vi "copy template project.vi"(8 "error in":errorcluster, 11 "project directory":path) -> (0 "error out":errorcluster)   [LabVIEW 2014, in "CD model script.lvlib"]
uses:
  CD model script.lvlib
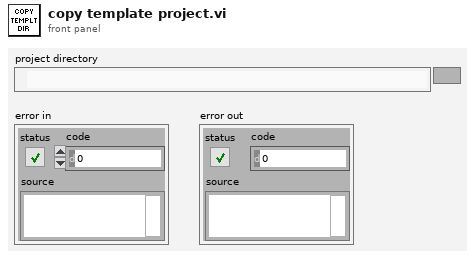
[diagram p1: front panel]
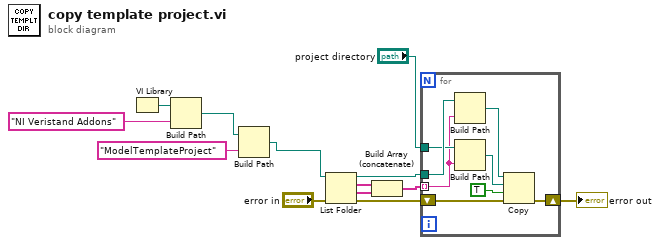
[diagram p0: block diagram]
diagram:
  n1 = VI Library() -> (path=w1:path)
  n2 = Build Path(base path=w1, name or relative path="NI Veristand Addons") -> (appended path=w3:path)
  n3 = Build Path(base path=w3, name or relative path="ModelTemplateProject") -> (appended path=w10:path)
  n4 = List Folder(path=w10, error in="error in") -> (path out=w8:path, filenames=w7:string[], folder names=w6:string[], error out=w9:errorcluster)  [unwired: 2 in]
  n5 = Build Array (concatenate)(w7, w6) -> (w5:string[])
  n6 = for {
    tunnel: "project directory" -> [w17]
    shift-right: [w20] -> w13
    shift-left: w9 -> [w21]
    tunnel: w8 -> [w18]
    tunnel: w5 -> [w16] mode=indexing
    n7 = Build Path(base path=w18, name or relative path=w16) -> (appended path=w14:path)
    n8 = Build Path(base path=w17, name or relative path=w16) -> (appended path=w15:path)
    n9 = Copy(8:w21, 9:TRUE ("overwrite (F)"), 10:w15, 11:w14) -> (0:w20:errorcluster)  [unwired: 1 in, 2 out]
  }
  "error out" <- w13
